vi "Constants.vi"() -> ()   [LabVIEW 2020, in "Waveform Analog Output Shared.lvlib"]
doc: "Use this Global VI to access the GUIDs assigned to the page resources of the Custom Device."
uses:
  Waveform Analog Output Shared.lvlib
panel:
  in  "Tab Control":T1(tab)=enum."Properties"
  in  "Status Page":string="0217cd2d-b942-4db7-90cc-07a95c7aaa37"
  in  "AO Parameter":string="55162da2-8447-4cd5-9327-959574672a6c"
  in  "AO Channel":string="96afaf3e-5a97-400f-9939-dce0822ed639"
  in  "Waveform Analog Output":string="b317c21f-b9d3-4af8-991e-248377f6c2c4"
  in  "Version Message":string="DAQ Waveform Generation Custom Device (ver 1.7) Started\n"
  in  "user.cd.#L2OutputBuffers":string="user.cd.#L1OutputBuffers"
  in  "user.cd.DataLoopUpdateIntervalms":string="user.cd.DataLoopUpdateIntervalms"
  in  "user.cd.#AOChannels":string="user.cd.#AOChannels"
  in  "user.cd.#L1OutputBuffers":string="user.cd.#L1OutputBuffers"
  in  "user.cd.StartDelay":string="user.cd.StartDelay"
  in  "user.cd.#Samples":string="user.cd.#Samples"
  in  "user.cd.PhysicalChannel":string="user.cd.PhysicalChannel"
  in  "user.cd.PhysicalChannels":string="user.cd.PhysicalChannels"
  in  "user.cd.DAQName":string="user.cd.DAQName"
  in  "user.cd.SampleRate":string="user.cd.SampleRate"
  in  "user.cd.MaxV":string="user.cd.MaxV"
  in  "user.cd.MinV":string="user.cd.MinV"
  out "Waveform Generation Error":errorcluster
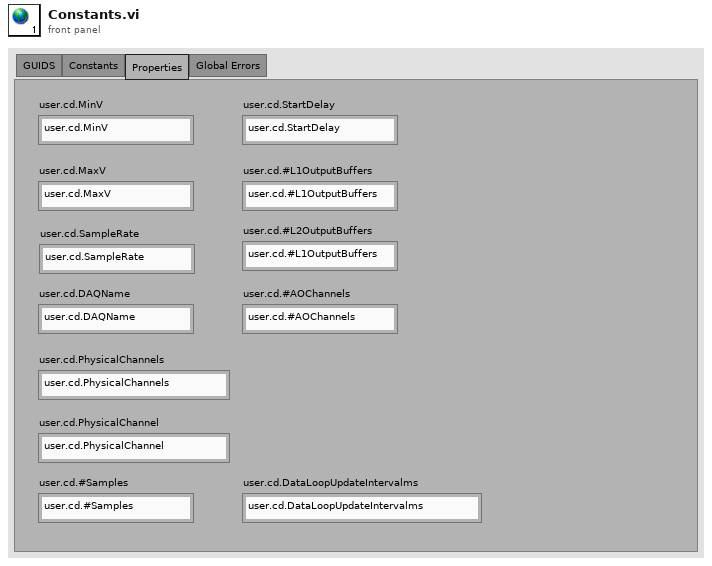
[diagram p1: front panel]
types:
  T1 = enum32{"GUIDS", "Constants", "Properties", "Global Errors"}
diagram:
